vi "download.vi"(8 "error in (no error)":errorcluster, 11 "plugin_interface in":refnum<class "odbc_driver_postgres_v13.0.2.lvclass">) -> (0 "error out":errorcluster, 3 "plugin_interface out":refnum<class "odbc_driver_postgres_v13.0.2.lvclass">)   [LabVIEW 2015, in "lv-example-postgres-post-installer.lvlib" / "odbc_driver_postgres_v13.0.2.lvclass"]
uses:
  odbc_driver_postgres_v13.0.2.lvclass
  <vilib>/Utility/error.llb/Error Cluster From Error Code.vi
  <vilib>/ErrorRing/Error Ring.xnode
  <userlib>/antonio-alexander/lv-bin-wget/public/api/v1/v1.lvlib
  <userlib>/antonio-alexander/lv-post-installer/lv-post-installer/lv-post-installer.lvlib
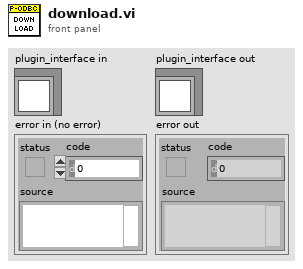
[diagram p1: front panel]
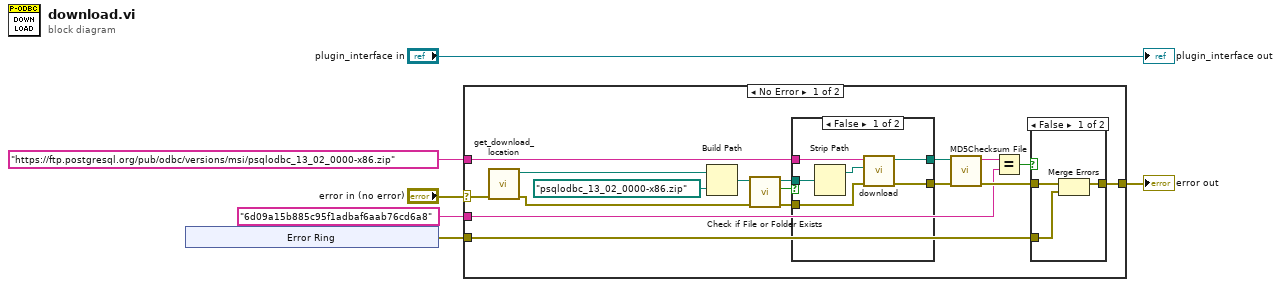
[diagram p0: block diagram]
diagram:
  n1 = xnode "Error Ring"() -> ("error out"=w6:errorcluster)
  n2 = case shown="No Error" "error in (no error)" {
    selector: "error in (no error)" -> [w10 w36]
    tunnel: "https://ftp.postgresql.org/pub/odbc/versions/msi/psqlodbc_13_02_0000-x86.zip" ("Download URL") -> [w23 _]
    tunnel: [w16 w36] -> w2
    tunnel: "6d09a15b885c95f1adbaf6aab76cd6a8" -> [w14 _]
    tunnel: w6 -> [w12 _]
    frame No Error {
      n3 = call <userlib>:"get_download_location.vi"("error in (no error)"=w10) -> ("error out"=w9:errorcluster, "download_location"=w11:path)  [unwired: 9 in]
      n4 = Build Path(base path=w11, name or relative path=path "psqlodbc_13_02_0000-x86.zip" ("appended path")) -> (appended path=w7:path)
      n5 = call <vilib>:"Check if File or Folder Exists.vi"("error in (no error)"=w9, "path"=w7) -> ("error out"=w22:errorcluster, "file or folder exists?"=w21:bool, "dup path"=w13:path)  [unwired: 7 in]
      n6 = case shown="False" w21 {
        tunnel: w23 -> [w29 _]
        tunnel: [w27 w31] -> w17
        tunnel: w22 -> [w24 w31]
        tunnel: [w28 w30] -> w15
        tunnel: w13 -> [w26 w30]
        frame False {
          n7 = Strip Path(path=w26) -> (stripped path=w25:path)  [unwired: 1 out]
          n8 = call <userlib>:"download.vi"("error in (no error)"=w24, "target_path"=w25, "address"=w29) -> ("error out"=w27:errorcluster, "filepath"=w28:path)  [unwired: 7 in]
        }
        frame True {
        }
      }
      n9 = call <vilib>:"MD5Checksum File.vi"("error in (no error)"=w17, "Path"=w15) -> ("error out"=w20:errorcluster, "MD5 message-digest"=w19:string)  [unwired: 8 in]
      n10 = Equal?(x=w19, y=w14) -> (x = y?=w18:bool)
      n11 = case shown="False" w18 {
        tunnel: w20 -> [w34 w35]
        tunnel: [w32 w35] -> w16
        tunnel: w12 -> [w33 _]
        frame False {
          n12 = Merge Errors(w34, w33) -> (w32:errorcluster)
        }
        frame True {
        }
      }
    }
    frame Error {
    }
  }
  "error out" <- w2
  "plugin_interface out" <- "plugin_interface in"
